vi "InspectExecuteCleanup.vi"(6 "Error":errorcluster, 7 "Actor":refnum<class "Actor.lvclass">, 10 "Msg":T6 {"MsgAttribs"."AbsoluteTime" format="%<%x %.3X>T"}, 11 "Actor":T1) -> (2 "Msg":T6 {"MsgAttribs"."AbsoluteTime" format="%<%x %.3X>T"}, 3 "Actor":T1, 4 "Error":errorcluster, 5 "Actor":refnum<class "Actor.lvclass">)   [LabVIEW 2020, in "jettl.lvlib" / "Actor.lvclass"]
uses:
  Actor.lvclass
  Msg/Msg.lvclass
  Metadata/Metadata.lvclass
  Origin.ctl
  jettl.lvlib
  Lifecycle.ctl
  MsgExecuteType.ctl
  MsgAttribs.ctl
  Msg.ctl
  PostSetup.ctl
  PreSetup.ctl
  MsgNames.ctl
  ActorAttribs.ctl
  ChildActors.ctl
  Actor.ctl
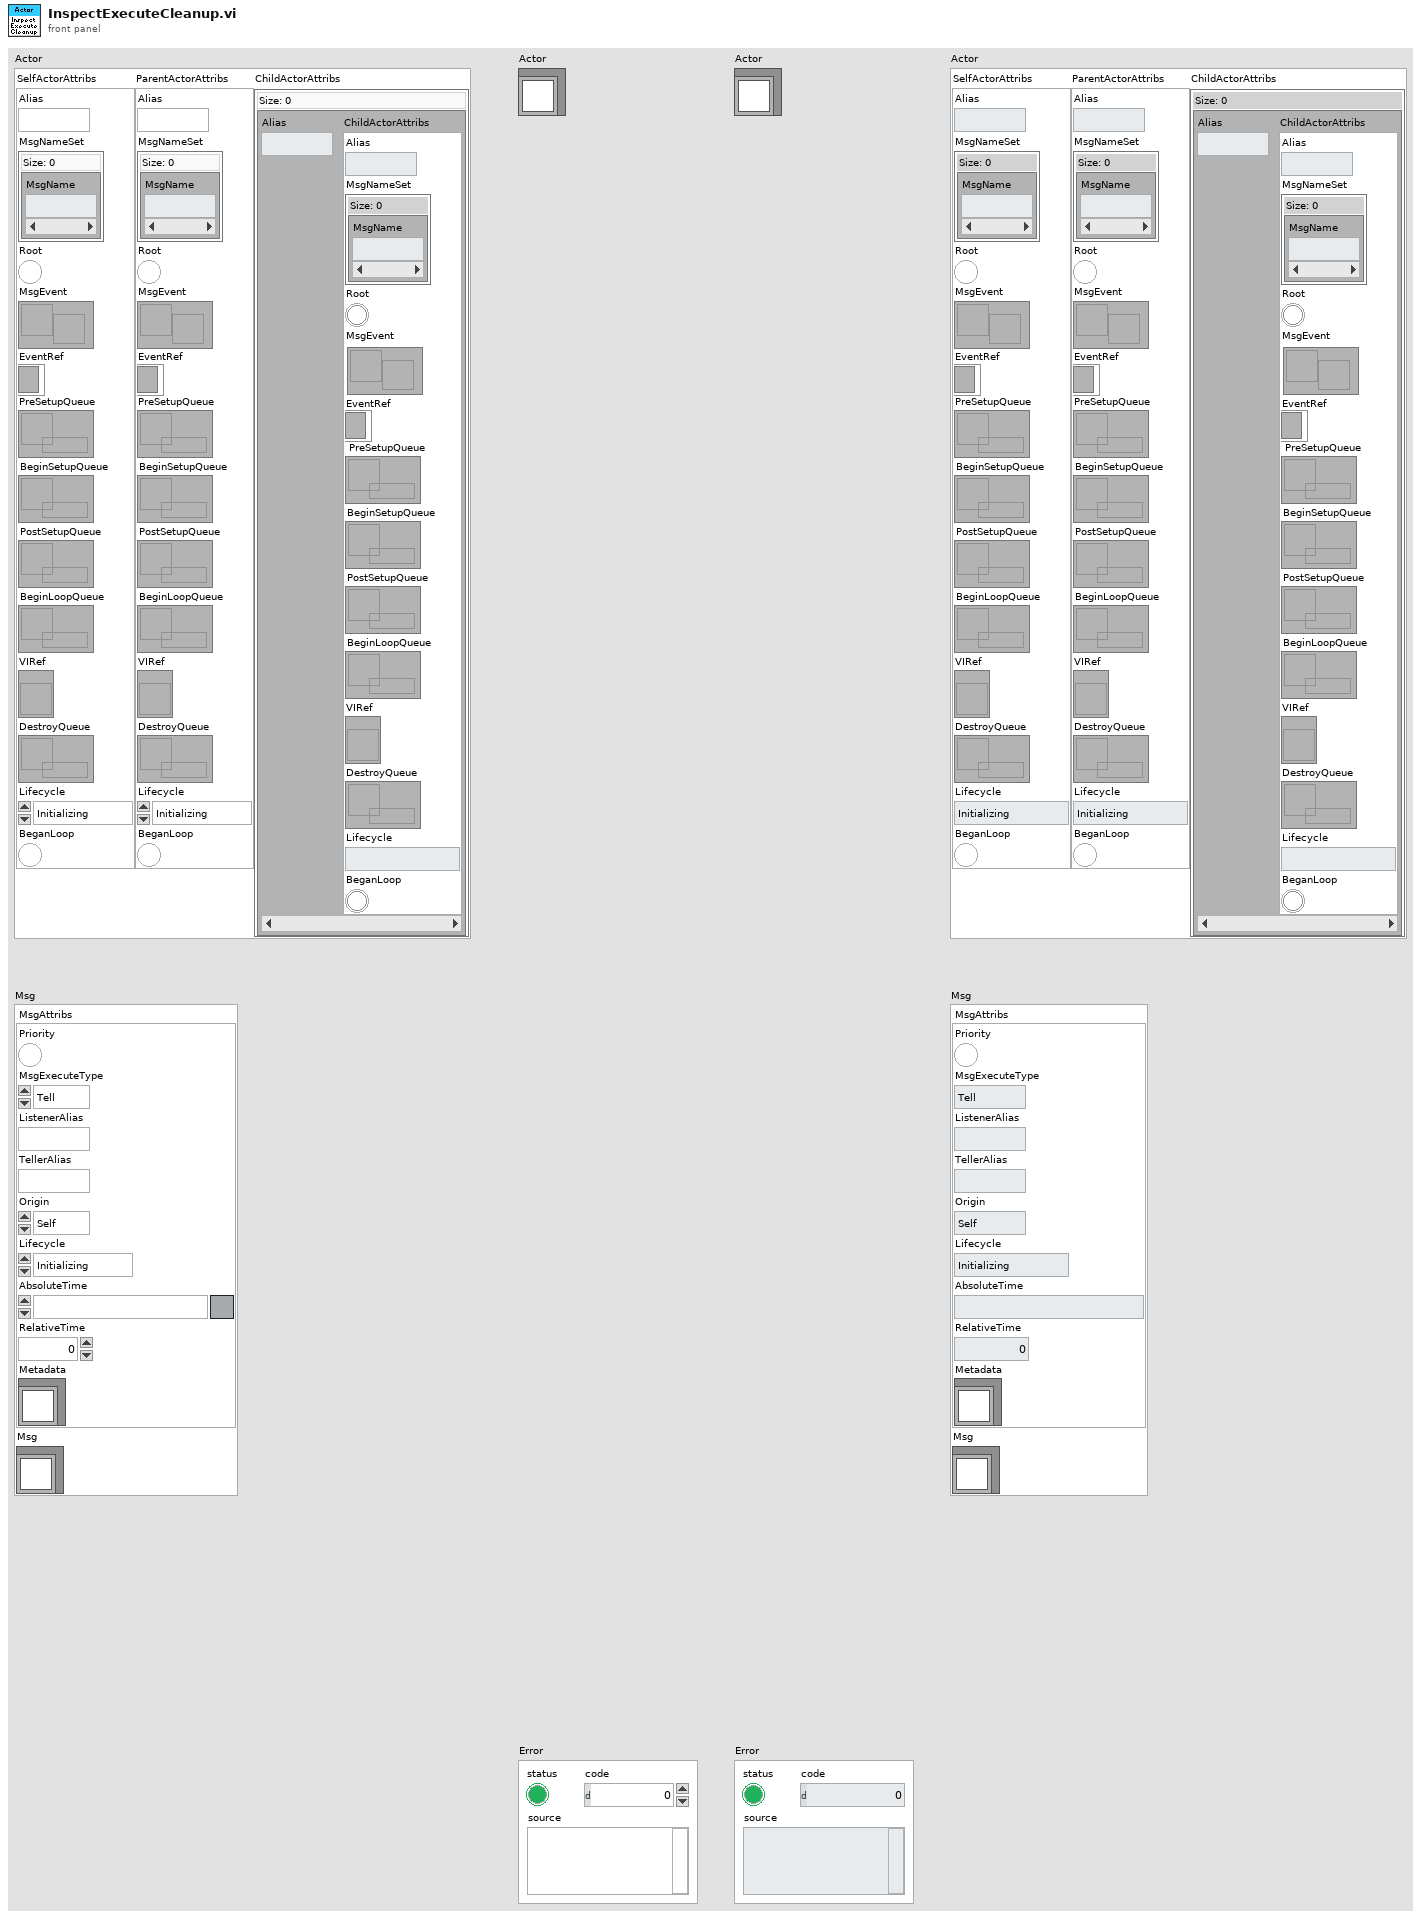
[diagram p1: front panel]
types:
  T1 = typedef "jettl.lvlib/Actor.ctl" = cluster{"SelfActorAttribs":T2, "ParentActorAttribs":T2, "ChildActorAttribs":T5}
  T2 = typedef "jettl.lvlib/ActorAttribs.ctl" = cluster{"Alias":string, "MsgNameSet":T3, "Root":bool, "MsgEvent":refnum<user-event>, "EventRef":refnum<event-registration>, "PreSetupQueue":refnum<queue>, "BeginSetupQueue":refnum<queue>, "PostSetupQueue":refnum<queue>, "BeginLoopQueue":refnum<queue>, "VIRef":refnum<vi>, "DestroyQueue":refnum<queue>, "Lifecycle":T4, "BeganLoop":bool}
  T3 = typedef "jettl.lvlib/MsgNames.ctl" = set{string}
  T4 = typedef "jettl.lvlib/Lifecycle.ctl" = enum16{"Initializing", "SettingUp", "Starting", "Running", "Stopping", "TearingDown", "Terminated"}
  T5 = typedef "jettl.lvlib/ChildActors.ctl" = map{string, T2}
  T6 = typedef "jettl.lvlib/Msg.ctl" = cluster{"MsgAttribs":T7, "Msg":refnum<class "Msg.lvclass">}
  T7 = typedef "jettl.lvlib/MsgAttribs.ctl" = cluster{"Priority":bool, "MsgExecuteType":T8, "ListenerAlias":string, "TellerAlias":string, "Origin":T9, "Lifecycle":T4, "AbsoluteTime":timestamp, "RelativeTime":dbl, "Metadata":refnum<class "Metadata.lvclass">}
  T8 = typedef "jettl.lvlib/MsgExecuteType.ctl" = enum16{"Tell", "Call"}
  T9 = typedef "jettl.lvlib/Origin.ctl" = enum16{"Self", "Parent", "Child"}
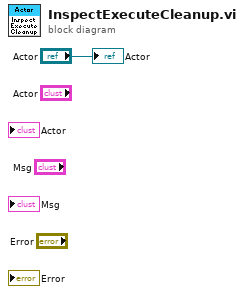
[diagram p0: block diagram]
diagram:
  "Actor" <- "Actor"
